vi "加标回收停止对话框.vi"() -> ()   [LabVIEW 2016, in "质控单元V4.lvlib"]
panel:
  in  "采配水":bool caption="启用"
  in  "取消":bool
  in  "确认":bool
  in  "CODCr":bool caption="启用"
  in  "CODMn":bool caption="启用"
  in  "总氮":bool caption="启用"
  in  "总磷":bool caption="启用"
  in  "氨氮":bool caption="启用"
  # "请选择要停止的参数"
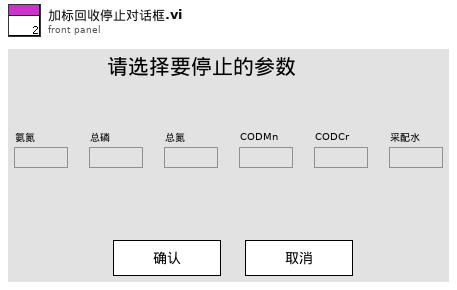
[diagram p1: front panel]
types:
  T1 = cluster{"氨氮":bool, "总磷":bool, "总氮":bool, "CODMn":bool, "CODCr":bool, "氨氮总磷":bool, "总磷总氮":bool}
  T2 = typedef "质控单元V4.lvlib/质控流程控制.ctl" = enum16{"待机", "启动进样流程", "启动加标流程", "启动排液流程", "启动润洗流程", "停止流程"}
  T3 = typedef "质控单元V4.lvlib/质控slave id.ctl" = enum16{"null", "氨氮", "总磷", "总氮", "CODMn", "CODCr", "氨氮总磷", "总磷总氮"}
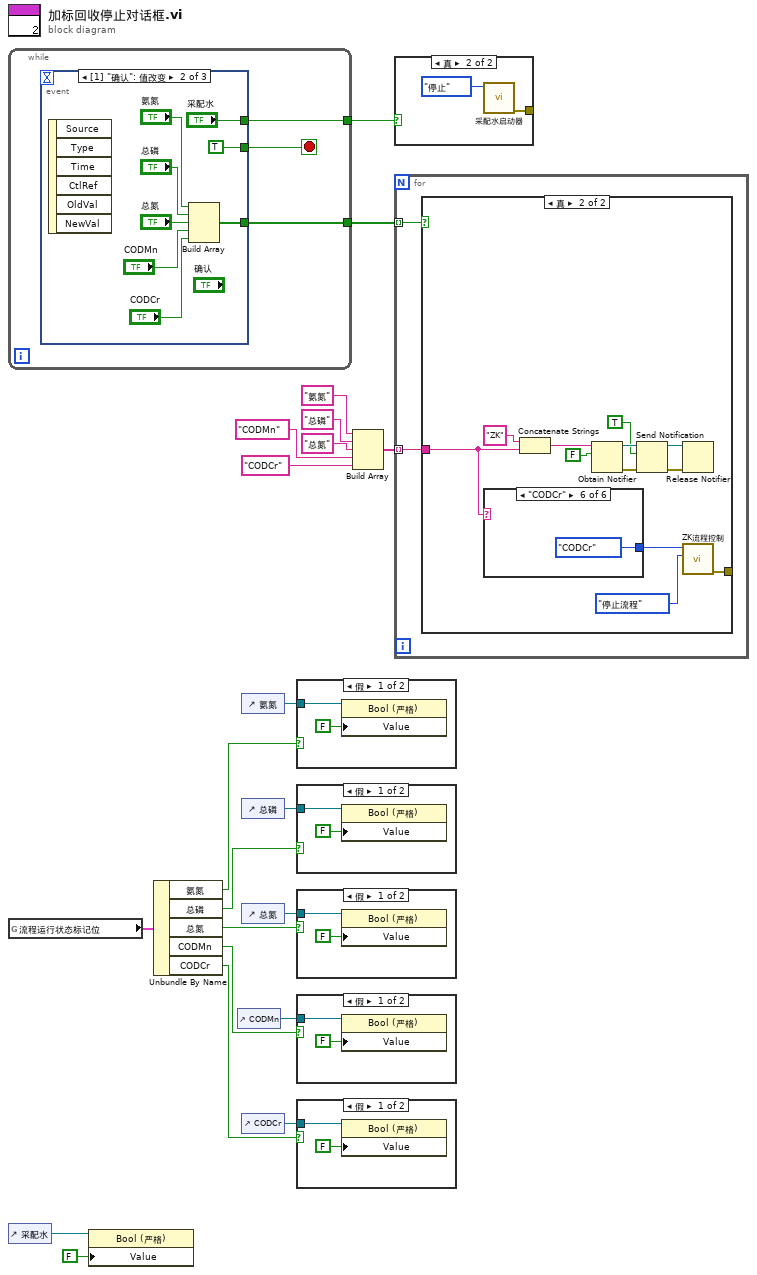
[diagram p0: block diagram]
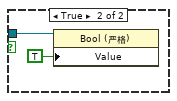
[diagram p3: hidden frame]
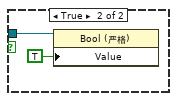
[diagram p4: hidden frame]
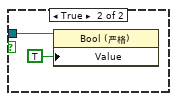
[diagram p5: hidden frame]
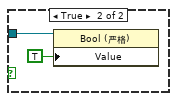
[diagram p6: hidden frame]
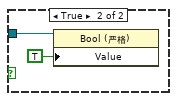
[diagram p7: hidden frame]
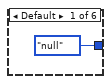
[diagram p9: hidden frame]
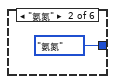
[diagram p10: hidden frame]
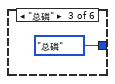
[diagram p11: hidden frame]
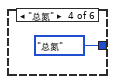
[diagram p12: hidden frame]
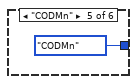
[diagram p13: hidden frame]
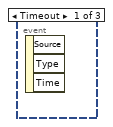
[diagram p14: hidden frame]
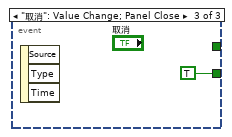
[diagram p15: hidden frame]
diagram:
  n1 = while {
    tunnel: [w23] -> w15
    tunnel: [w22] -> w3
    stop <- w24 stop-if-true
    n2 = event shown="[1] \"确认\": 值改变" {
      selector: _ -> [_ _ _]
      dyn-events: _ -> [_ _ _]
      timeout: _ -> [_ _ _]
      tunnel: [_ TRUE TRUE] -> w24
      tunnel: [_ w26 _] -> w23
      tunnel: [_ "采配水" _] -> w22
      event Timeout {
        n3 = event-data() -> ()  [unwired: 1 in, 3 out]
      }
      event "确认": Value Change {
        n4 = event-data() -> ()  [unwired: 1 in, 6 out]
        n5 = Build Array("氨氮", "总磷", "总氮", "CODMn", "CODCr") -> (w26:bool[])
      }
      event "取消": Value Change; Panel Close {
        n6 = event-data() -> ()  [unwired: 1 in, 3 out]
      }
    }
  }
  n7 = global read "ZK非断电保存全局变量.vi" "流程运行状态标记位"() -> (w14:T1)
  n8 = control-ref of="采配水"() -> (w1:refnum<vi>)
  n9 = property class="Bool (严格)"(reference=w1, "Value"=FALSE ("值")) -> ()  [unwired: 1 in, 2 out]
  n10 = Unbundle By Name(w14) -> ("氨氮"=w13:bool, "总磷"=w12:bool, "总氮"=w11:bool, "CODMn"=w10:bool, "CODCr"=w9:bool)
  n11 = control-ref of="CODMn"() -> (w5:refnum<vi>)
  n12 = control-ref of="氨氮"() -> (w8:refnum<vi>)
  n13 = control-ref of="总磷"() -> (w7:refnum<vi>)
  n14 = control-ref of="总氮"() -> (w6:refnum<vi>)
  n15 = control-ref of="CODCr"() -> (w4:refnum<vi>)
  n16 = case shown="假" w13 {
    tunnel: w8 -> [w35 w37]
    frame False {
      n17 = property class="Bool (严格)"(reference=w35, "Value"=FALSE ("值")) -> ()  [unwired: 1 in, 2 out]
    }
    frame True {
      n18 = property class="Bool (严格)"(reference=w37, "Value"=TRUE ("值")) -> ()  [unwired: 1 in, 2 out]
    }
  }
  n19 = case shown="假" w12 {
    tunnel: w7 -> [w39 w41]
    frame False {
      n20 = property class="Bool (严格)"(reference=w39, "Value"=FALSE ("值")) -> ()  [unwired: 1 in, 2 out]
    }
    frame True {
      n21 = property class="Bool (严格)"(reference=w41, "Value"=TRUE ("值")) -> ()  [unwired: 1 in, 2 out]
    }
  }
  n22 = case shown="假" w11 {
    tunnel: w6 -> [w43 w45]
    frame False {
      n23 = property class="Bool (严格)"(reference=w43, "Value"=FALSE ("值")) -> ()  [unwired: 1 in, 2 out]
    }
    frame True {
      n24 = property class="Bool (严格)"(reference=w45, "Value"=TRUE ("值")) -> ()  [unwired: 1 in, 2 out]
    }
  }
  n25 = case shown="假" w10 {
    tunnel: w5 -> [w47 w49]
    frame False {
      n26 = property class="Bool (严格)"(reference=w47, "Value"=FALSE ("值")) -> ()  [unwired: 1 in, 2 out]
    }
    frame True {
      n27 = property class="Bool (严格)"(reference=w49, "Value"=TRUE ("值")) -> ()  [unwired: 1 in, 2 out]
    }
  }
  n28 = case shown="假" w9 {
    tunnel: w4 -> [w51 w53]
    frame False {
      n29 = property class="Bool (严格)"(reference=w51, "Value"=FALSE ("值")) -> ()  [unwired: 1 in, 2 out]
    }
    frame True {
      n30 = property class="Bool (严格)"(reference=w53, "Value"=TRUE ("值")) -> ()  [unwired: 1 in, 2 out]
    }
  }
  n31 = Build Array("氨氮", "总磷", "总氮", "CODMn", "CODCr") -> (w16:string[])
  n32 = case shown="真" w3 {
    tunnel: [_ w54] -> _
    frame False {
    }
    frame True {
      n33 = call "采配水启动器.vi"("启动/停止命令"=enum16{"待机", "水样测试", "停止", "加标回收"}."停止") -> ("error out"=w54:errorcluster)  [unwired: 10 in]
    }
  }
  n34 = for {
    tunnel: w16 -> [w57] mode=indexing
    tunnel: w15 -> [w56] mode=indexing
    n35 = case shown="真" w56 {
      tunnel: w57 -> [_ w60]
      tunnel: [_ w58] -> _
      frame False {
      }
      frame True {
        n36 = case shown="\"CODCr\"" w60 {
          tunnel: [质控slave_id."null" ("Slave ID") 质控slave_id."氨氮" ("Slave ID") 质控slave_id."总磷" ("Slave ID") 质控slave_id."总氮" ("Slave ID") 质控slave_id."CODMn" ("Slave ID") 质控slave_id."CODCr" ("Slave ID")] -> w59
          frame Default {
          }
          frame "氨氮" {
          }
          frame "总磷" {
          }
          frame "总氮" {
          }
          frame "CODMn" {
          }
          frame "CODCr" {
          }
        }
        n37 = Concatenate Strings("ZK" ("名称（未命名）"), w60) -> (w67:string)
        n38 = Obtain Notifier(name (unnamed)=w67, notification data type=FALSE) -> (notifier out=w66:refnum<notifier>, error out=w65:errorcluster)  [unwired: 2 in, 1 out]
        n39 = Send Notification(notification=TRUE ("通知"), notifier=w66, error in (no error)=w65) -> (notifier out=w64:refnum<notifier>, error out=w63:errorcluster)
        n40 = Release Notifier(notifier=w64, error in (no error)=w63) -> ()  [unwired: 1 in, 3 out]
        n41 = call "ZK流程控制.vi"("流程控制"=质控流程控制."停止流程", "Slave ID"=w59) -> ("error out"=w58:errorcluster)  [unwired: 9 in]
      }
    }
  }
